vi "Check User Pin.vi"(8 "error in (no error)":errorcluster, 10 "User Pin":string, 11 "ATM Data":T1={"UI Refs"={"Right Buttons"=refnum, "Left Buttons"=refnum, "User Input"=refnum, "ATM Messages"=refnum, "Left Menu"=refnum, "Right Menu"=refnum, "Enter"=refnum}, "Map"={}, "Login Valid?"=FALSE, "Queue Message"=refnum, "State"=enum."None", "User"={"Pin"="", "First Name"="", "Last Name"="", "Balance"=0.0, "Login Valid?"=FALSE}, "Main States"={"Message"="Initialize", "Data"=variant}}) -> (0 "error out":errorcluster, 3 "ATM Data Out":T1={"UI Refs"={"Right Buttons"=refnum, "Left Buttons"=refnum, "User Input"=refnum, "ATM Messages"=refnum, "Left Menu"=refnum, "Right Menu"=refnum, "Enter"=refnum}, "Map"={}, "Login Valid?"=FALSE, "Queue Message"=refnum, "State"=enum."None", "User"={"Pin"="", "First Name"="", "Last Name"="", "Balance"=0.0, "Login Valid?"=FALSE}, "Main States"={"Message"="Initialize", "Data"=variant}})   [LabVIEW 2020, in "ATM Machine.lvlib"]
uses:
  ATM Machine.lvlib
  Cluster - ATM Machine Data.ctl
  Cluster - Message Cluster.ctl
  Enum - ATM States.ctl
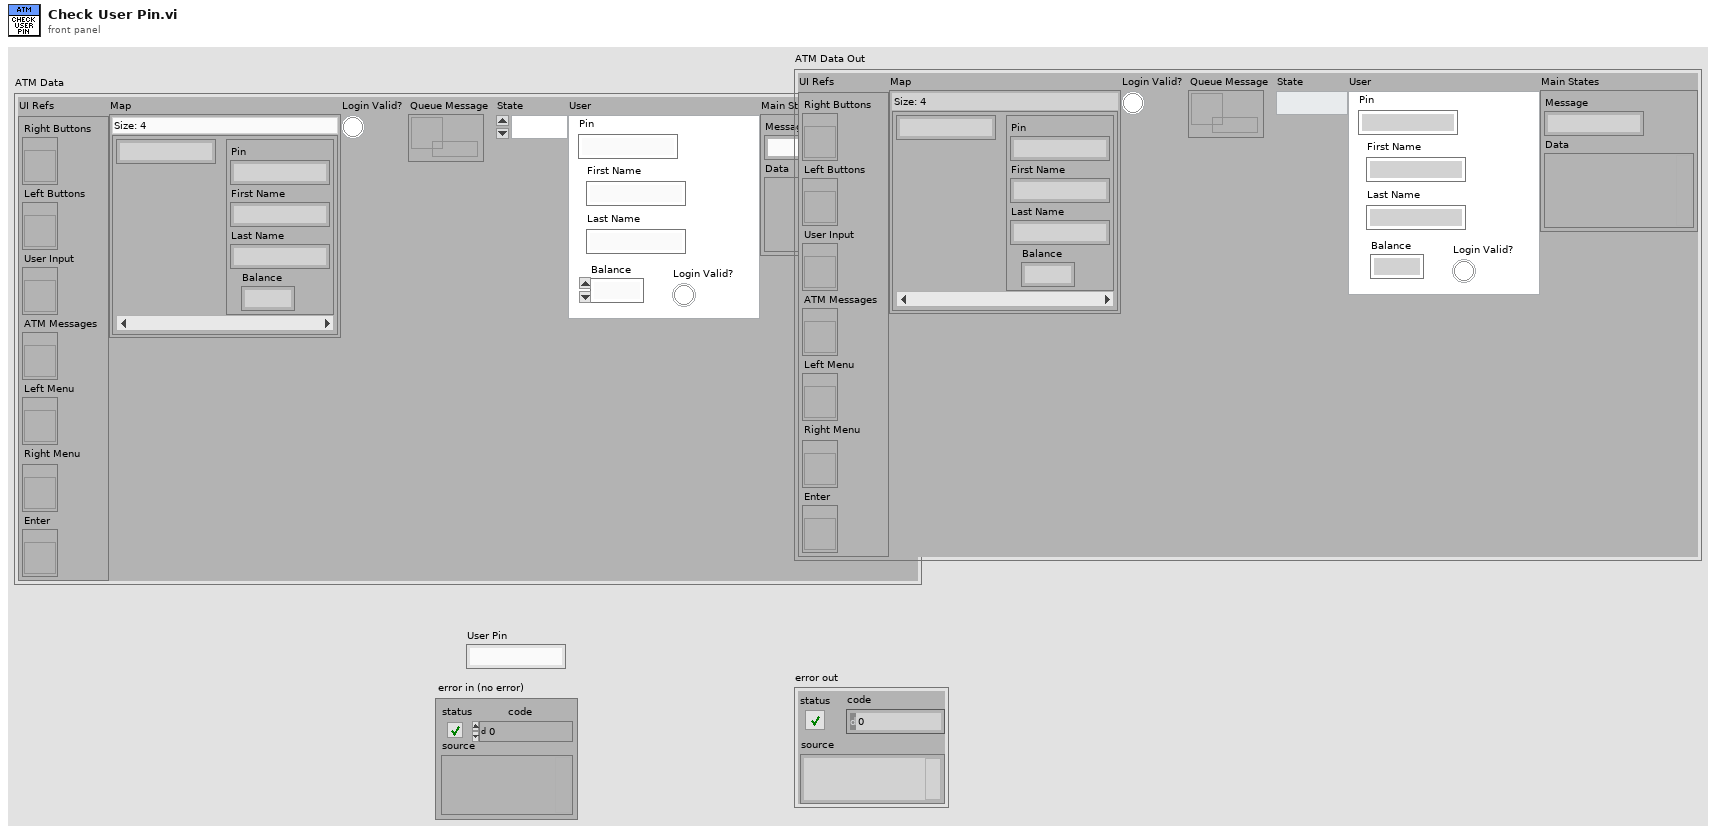
[diagram p1: front panel]
types:
  T1 = typedef "ATM Machine.lvlib/Cluster - ATM Machine Data.ctl" = cluster{"UI Refs":cluster{"Right Buttons":refnum<vi>, "Left Buttons":refnum<vi>, "User Input":refnum<vi>, "ATM Messages":refnum<vi>, "Left Menu":refnum<vi>, "Right Menu":refnum<vi>, "Enter":refnum<vi>}, "Map":map{string, cluster{"Pin":string, "First Name":string, "Last Name":string, "Balance":dbl}}, "Login Valid?":bool, "Queue Message":refnum<queue>, "State":T2, "User":cluster{"Pin":string, "First Name":string, "Last Name":string, "Balance":dbl, "Login Valid?":bool}, "Main States":cluster{"Message":string, "Data":variant}}
  T2 = typedef "ATM Machine.lvlib/Enum - ATM States.ctl" = enum16{"None", "Deposit", "Withdraw", "Card Inserted", "Balance Inquiry", "Return Card and Terminate", "Fast Cash"}
  T3 = map{string, cluster{"Pin":string, "First Name":string, "Last Name":string, "Balance":dbl}}
  T4 = cluster{"Pin":string, "First Name":string, "Last Name":string, "Balance":dbl}
  T5 = enum8{"Enabled", "Disabled", "Disabled and Grayed Out"}
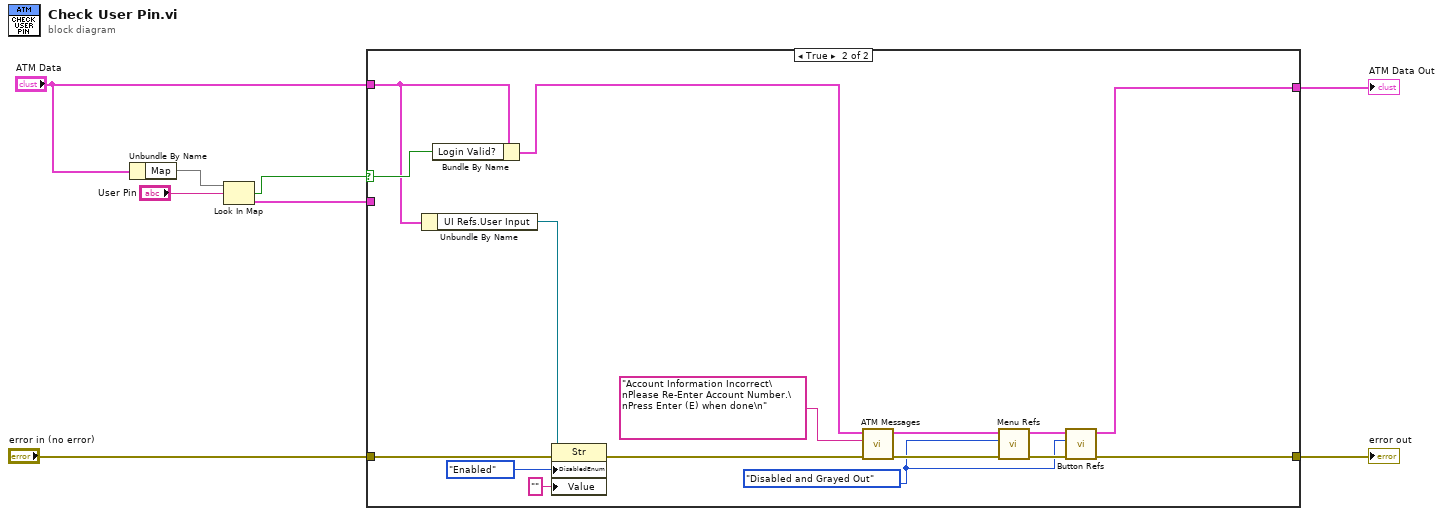
[diagram p0: block diagram]
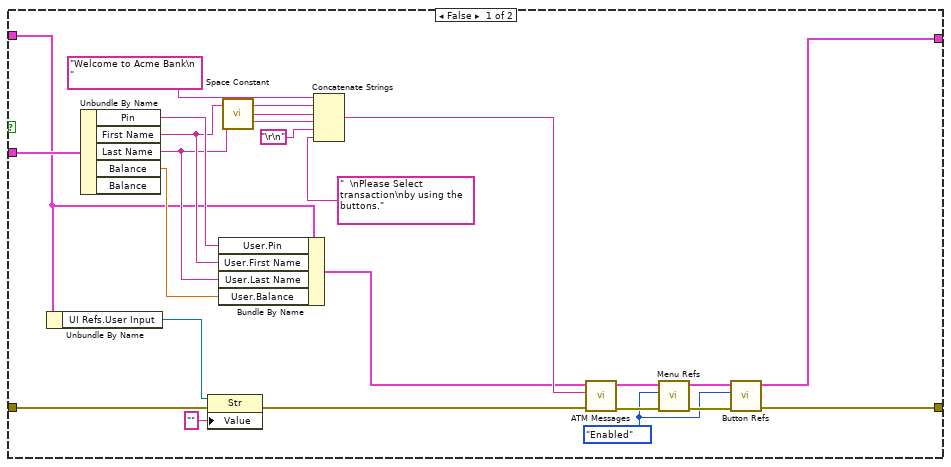
[diagram p2: hidden frame]
diagram:
  n1 = Unbundle By Name("ATM Data") -> ("Map"=w2:T3)
  n2 = Look In Map(map=w2, key="User Pin") -> (key not found?=w5:bool, value=w1:T4)  [unwired: 1 in]
  n3 = case shown="True" w5 {
    selector: w5 -> [_ w36]
    tunnel: [w22 w43] -> w8
    tunnel: "error in (no error)" -> [w11 w38]
    tunnel: w1 -> [w30 _]
    tunnel: "ATM Data" -> [w13 w34]
    tunnel: [w19 w33] -> w3
    frame False {
      w21 = T5."Enabled" ("Disabled 2")
      n4 = Unbundle By Name(w13) -> ("UI Refs.User Input"=w9:refnum<vi>)
      n5 = Unbundle By Name(w30) -> ("Pin"=w18:string, "First Name"=w17:string, "Last Name"=w16:string, "Balance"=w15:dbl)  [unwired: 1 out]
      n6 = property class="Str"(reference=w9, error in=w11, "Value"="") -> (error out=w12:errorcluster)  [unwired: 1 out]
      n7 = Bundle By Name(cluster=w13, "User.Pin"=w18, "User.First Name"=w17, "User.Last Name"=w16, "User.Balance"=w15) -> (w14:T1)
      n8 = call <vilib>:"Space Constant.vi"() -> ("String"=w28:string)
      n9 = Concatenate Strings("Welcome to Acme Bank\n   " ("string"), w17, w28, w16, "\r\n", "  \nPlease Select transaction\nby using the buttons." ("string")) -> (w29:string)
      n10 = call "ATM Messages.vi"("error in"=w12, "ATM Message"=w29, "ATM Data"=w14) -> ("error out"=w25:errorcluster, "ATM Data Out"=w24:T1)  [unwired: 7 in]
      n11 = call "Menu Refs.vi"("error in"=w25, "Disabled 2"=w21, "ATM Data"=w24) -> ("error out"=w23:errorcluster, "ATM Data Out"=w20:T1)  [unwired: 7 in]
      n12 = call "Button Refs.vi"("error in"=w23, "Disabled"=w21, "ATM Data"=w20) -> ("error out"=w22:errorcluster, "ATM Data Out"=w19:T1)  [unwired: 7 in]
    }
    frame True {
      w41 = T5."Disabled and Grayed Out" ("Disabled 2")
      n13 = Unbundle By Name(w34) -> ("UI Refs.User Input"=w40:refnum<vi>)
      n14 = Bundle By Name(cluster=w34, "Login Valid?"=w36) -> (w35:T1)
      n15 = property class="Str"(reference=w40, error in=w38, "DisabledEnum"=T5."Enabled" ("Disabled"), "Value"="") -> (error out=w39:errorcluster)  [unwired: 1 out]
      n16 = call "ATM Messages.vi"("error in"=w39, "ATM Message"="Account Information Incorrect\nPlease Re-Enter Account Number.\nPress Enter (E) when done\n", "ATM Data"=w35) -> ("error out"=w46:errorcluster, "ATM Data Out"=w45:T1)  [unwired: 7 in]
      n17 = call "Menu Refs.vi"("error in"=w46, "Disabled 2"=w41, "ATM Data"=w45) -> ("error out"=w44:errorcluster, "ATM Data Out"=w42:T1)  [unwired: 7 in]
      n18 = call "Button Refs.vi"("error in"=w44, "Disabled"=w41, "ATM Data"=w42) -> ("error out"=w43:errorcluster, "ATM Data Out"=w33:T1)  [unwired: 7 in]
    }
  }
  "error out" <- w8
  "ATM Data Out" <- w3
